vi "Hold.vi"(8 "error in (no error)":errorcluster, 11 "PS Driver.lvlib:PS Driver.lvclass in":refnum<class "PS Driver.lvclass">) -> (0 "error out":errorcluster, 3 "PS Driver.lvlib:PS Driver.lvclass out":refnum<class "PS Driver.lvclass">)   [LabVIEW 2020, in "PS Driver.lvlib" / "PS Driver.lvclass"]
uses:
  PS Driver.lvclass
  PS Driver.lvclass/PS Driver.ctl
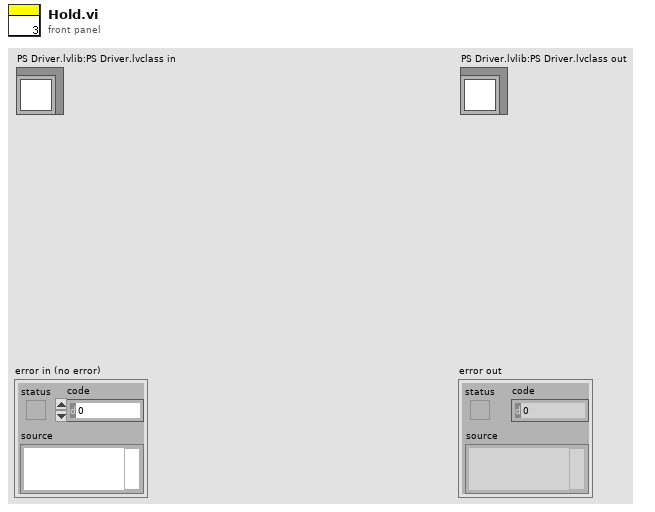
[diagram p1: front panel]
types:
  T1 = enum16{"Hold", "Ramp to zero", "Ramp to setpoint"}
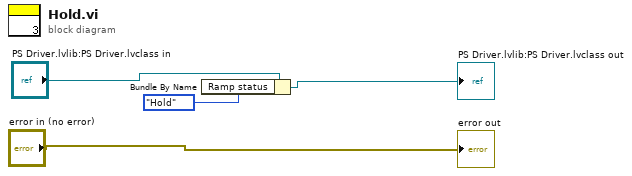
[diagram p0: block diagram]
diagram:
  n1 = Bundle By Name(cluster="PS Driver.lvlib:PS Driver.lvclass in", "Ramp status"=T1."Hold") -> (→"PS Driver.lvlib:PS Driver.lvclass out":refnum<class "PS Driver.lvclass">)
  "error out" <- "error in (no error)"
